vi "request.Read jsonrpc.vi"(8 "error in (no error)":errorcluster, 11 "Request in":refnum<class "Request.lvclass">) -> (0 "error out":errorcluster, 2 "jsonrpc":string, 3 "Request out":refnum<class "Request.lvclass">)   [LabVIEW 2020, in "JSON-RPC Lib.lvlib" / "Request.lvclass"]
uses:
  Request.lvclass
  Request.lvclass/Request.ctl
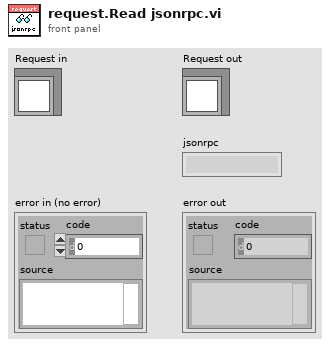
[diagram p1: front panel]
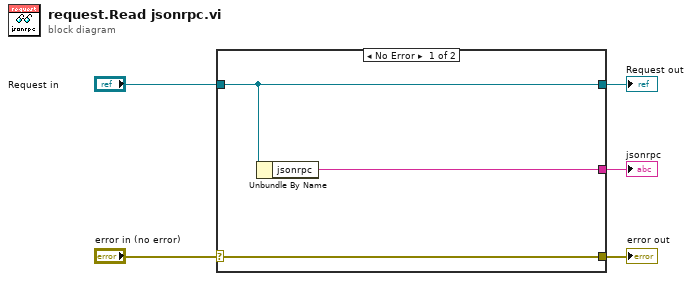
[diagram p0: block diagram]
diagram:
  n1 = case shown="No Error" "error in (no error)" {
    selector: "error in (no error)" -> [w8 w9]
    tunnel: [w8 w9] -> w4
    tunnel: [w7 w10] -> w2
    tunnel: "Request in" -> [w7 w10]
    tunnel: [w6 _] -> w1
    frame No Error {
      n2 = Unbundle By Name(w7) -> ("jsonrpc"=w6:string)
    }
    frame Error {
    }
  }
  "error out" <- w4
  "Request out" <- w2
  "jsonrpc" <- w1
